vi "SMO.UI.ByRefWithEvents.GetPublicEventsRegistration.vi"(8 "error in (no error)":errorcluster, 11 "SMO.UI.ByRefWithEvents":refnum<class "SMO.UI.ByRefWithEvents.lvclass">) -> (0 "error out":errorcluster, 2 "SMO.Template Public Events":refnum<event-registration>, 3 "SMO.UI.ByRefWithEvents out":refnum<class "SMO.UI.ByRefWithEvents.lvclass">)   [LabVIEW 2013, in "SMO.UI.ByRefWithEvents.lvclass"]
doc: "---------------------------------------------------------------\nJKI State Machine Objects™\nhttp://jki.net/state-machine-objects/\nCopyright (C) 2005-2015, JKI <info@jki.net>\nALL RIGHTS RESERVEDJKI State Machine Objects (SMO) 1.0.0.5\nJKI - JKI\nCopyright (c) 2016, JKI"
uses:
  SMO.UI.ByRefWithEvents.lvclass
  Typedefs/PublicEvents--Cluster.ctl
  Typedefs/DataChanged--EventData--Cluster.ctl
panel:
  # "For instructions on how to use the JKI State Machine Objects, examples and video tutorials, visit:\nhttp://jki.net/state-machine-objects/\n\nJKI State Machine Objects™\nhttp://jki.net/state-machine-objects/\nCopyright (C) 2005-2015, JKI <info@jki.net>\nALL RIGHTS RESERVED"
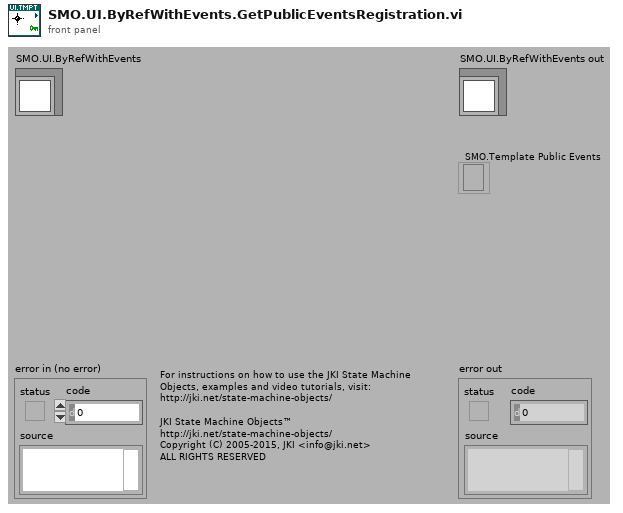
[diagram p1: front panel]
types:
  T1 = typedef "SMO.UI.ByRefWithEvents.lvclass/PublicEvents--Cluster.ctl" = cluster{"Data Changed":refnum<user-event>}
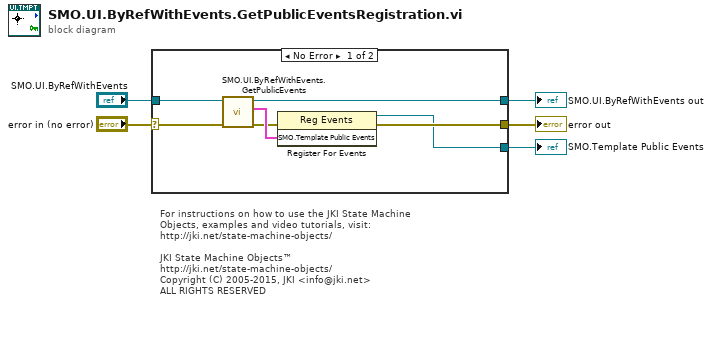
[diagram p0: block diagram]
diagram:
  # "For instructions on how to use the JKI State Machine Objects, examples and video tutorials, visit:\nhttp://jki.net/state-machine-objects/\n\nJKI State Machine Objects™\nhttp://jki.net/state-machine-objects/\nCopyright (C) 2005-2015, JKI <info@jki.net>\nALL RIGHTS RESERVED"
  n1 = case shown="No Error" "error in (no error)" {
    selector: "error in (no error)" -> [w6 w13]
    tunnel: "SMO.UI.ByRefWithEvents" -> [w11 w14]
    tunnel: [w9 w13] -> w4
    tunnel: [w10 w14] -> w3
    tunnel: [w8 _] -> w1
    frame No Error {
      n2 = call "SMO.UI.ByRefWithEvents.GetPublicEvents.vi"("error in (no error)"=w6, "SMO.UI.ByRefWithEvents"=w11) -> ("error out"=w7:errorcluster, "SMO.Template Public Events"=w12:T1, "SMO.UI.ByRefWithEvents out"=w10:refnum<class "SMO.UI.ByRefWithEvents.lvclass">)  [unwired: 7 in]
      n3 = register-events(error in=w7, w12) -> (reference out=w8:refnum<event-registration>, error out=w9:errorcluster)  [unwired: 1 in]
    }
    frame Error {
    }
  }
  "error out" <- w4
  "SMO.UI.ByRefWithEvents out" <- w3
  "SMO.Template Public Events" <- w1
